vi "Get TXP Results.vi"(8 "error in (no error)":errorcluster, 11 "niDTS BT INSTR TX in":refnum<class "niDTS BT INSTR TX.lvclass">) -> (0 "error out":errorcluster, 2 "output cluster":T1, 3 "niDTS BT INSTR TX out":refnum<class "niDTS BT INSTR TX.lvclass">)   [LabVIEW 2015, in "niDTS BT.lvlib" / "niDTS BT INSTR TX.lvclass"]
uses:
  niDTS BT INSTR TX.lvclass
  Tests/Tx Test/Includes/niDTS BT Tx Test INC TXP Results.ctl
  niDTS BT INSTR TX.lvclass/niDTS BT INSTR TX.ctl
  RiviInstDriver/niRfsaBT/Objects/niRfsaBt.lvclass
  niDTS BT.lvlib
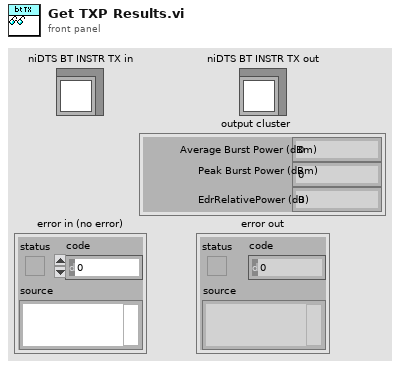
[diagram p1: front panel]
types:
  T1 = typedef "niDTS BT.lvlib/niDTS BT Tx Test INC TXP Results.ctl" = cluster{"Average Burst Power (dBm)":dbl, "Peak Burst Power (dBm)":dbl, "EdrRelativePower (dB)":dbl}
  T2 = cluster{"AverageBrustPower":dbl, "PeakBrustPower":dbl, "EdrRelativePower":dbl}
  T3 = typedef "niRfsaBT.lvclass/niRfsaBT INC Handle.ctl" = refnum<data-value>
  T4 = cluster{"AverageBurstPower":dbl, "AveragePeakBurstPower":dbl, "EdrRelativePower":dbl}
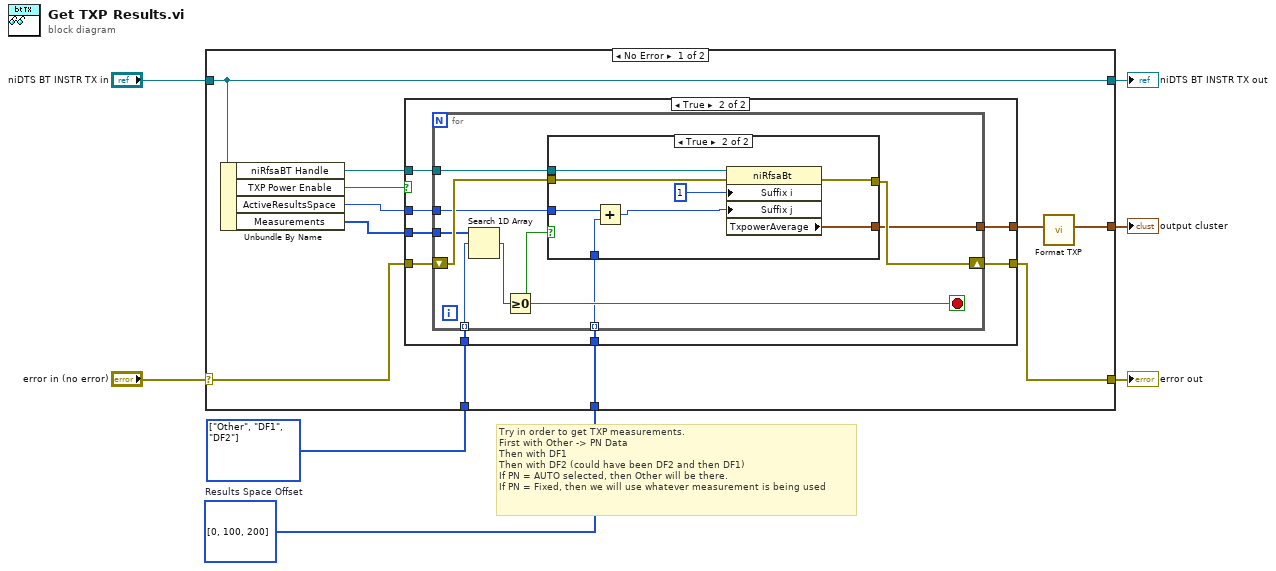
[diagram p0: block diagram]
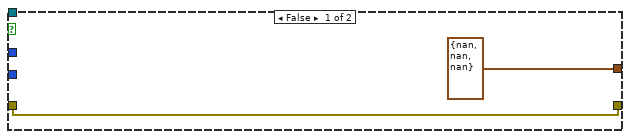
[diagram p2: hidden frame]
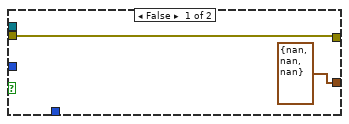
[diagram p3: hidden frame]
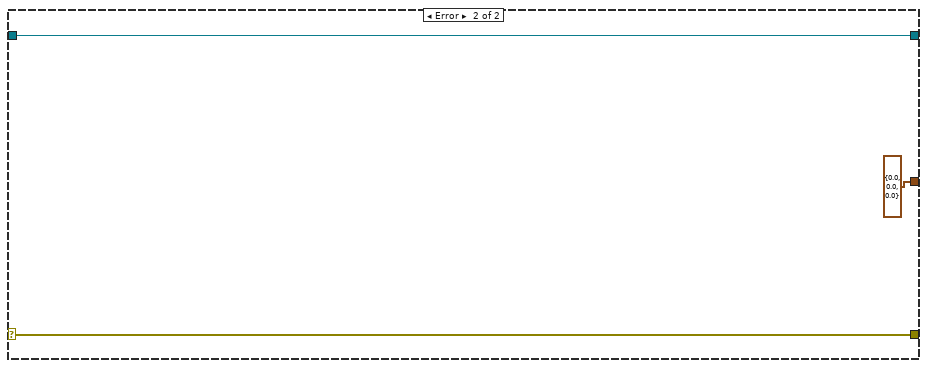
[diagram p4: hidden frame]
diagram:
  w1 = i32[] [0, 100, 200]  # Results Space Offset
  w2 = enum16{"Other", "DF1", "DF2"}[] [enum."Other", enum."DF1", enum."DF2"] items=["Other", "DF1", "DF2"] ("Measurements")
  # "Try in order to get TXP measurements.\nFirst with Other -> PN Data\nThen with DF1\nThen with DF2 (could have been DF2 and then DF1)\nIf PN = AUTO selected, then Other will be there.\nIf PN = Fixed, then we will use whatever measurement is being used"
  n1 = case shown="No Error" "error in (no error)" {
    selector: "error in (no error)" -> [w15 w50]
    tunnel: [w14 w50] -> w6
    tunnel: [w16 w51] -> w4
    tunnel: "niDTS BT INSTR TX in" -> [w16 w51]
    tunnel: [w13 T1 {"Average Burst Power (dBm)"=0.0, "Peak Burst Power (dBm)"=0.0, "EdrRelativePower (dB)"=0.0} ("output cluster")] -> w3
    tunnel: w2 -> [w9 _]
    tunnel: w1 -> [w8 _]
    frame No Error {
      n2 = Unbundle By Name(w16) -> ("niRfsaBT Handle"=w18:T3, "TXP Power Enable"=w17:bool, "ActiveResultsSpace"=w11:u8, "Measurements"=w10:enum16{"Other", "DF1", "DF2"}[])
      n3 = case shown="True" w17 {
        tunnel: w18 -> [_ w28]
        tunnel: w15 -> [w19 w27]
        tunnel: [w19 w26] -> w14
        tunnel: [T2 {"AverageBrustPower"=nan, "PeakBrustPower"=nan, "EdrRelativePower"=nan} ("[AVERage]_B") w25] -> w12
        tunnel: w11 -> [_ w24]
        tunnel: w10 -> [_ w23]
        tunnel: w9 -> [_ w22]
        tunnel: w8 -> [_ w21]
        frame False {
        }
        frame True {
          n4 = for {
            tunnel: w28 -> [w38]
            tunnel: [w35] -> w25
            tunnel: w24 -> [w34]
            tunnel: w23 -> [w31]
            shift-right: [w36] -> w26
            shift-left: w27 -> [w37]
            tunnel: w22 -> [w32] mode=indexing
            tunnel: w21 -> [w29] mode=indexing
            stop <- w30 stop-if-true
            n5 = Search 1D Array(1D array=w31, element=w32) -> (index of element=w33:i32)  [unwired: 1 in]
            n6 = Greater Or Equal To 0?(x=w33) -> (x >= 0?=w30:bool)
            n7 = case shown="True" w30 {
              tunnel: w38 -> [_ w48]
              tunnel: w37 -> [w40 w47]
              tunnel: [w40 w44] -> w36
              tunnel: [T2 {"AverageBrustPower"=nan, "PeakBrustPower"=nan, "EdrRelativePower"=nan} ("[AVERage]_B") w46] -> w35
              tunnel: w34 -> [_ w43]
              tunnel: w29 -> [_ w42]
              frame False {
              }
              frame True {
                n8 = Add(x=w43, y=w42) -> (x+y=w41:i32)
                n9 = property class="niRfsaBt"(reference=w48, error in=w47, "Suffix i"=1 ("Active Channel:Suffix i"), "Suffix j"=w41) -> (error out=w44:errorcluster, "TxpowerAverage"=w46:T4)  [unwired: 1 out]
              }
            }
          }
        }
      }
      n10 = call "Format TXP.vi"("TxP Results"=w12) -> ("Txp Results"=w13:T1)  [unwired: 10 in]
    }
    frame Error {
    }
  }
  "error out" <- w6
  "niDTS BT INSTR TX out" <- w4
  "output cluster" <- w3
